vi "Get Segments.vi"(8 "error in (no error)":errorcluster, 9 "Pct-Encoded? (F)":bool, 11 "URI-Component.Path in":refnum<class "URI-Component.Path.lvclass">) -> (0 "error out":errorcluster, 2 "Segments":string[](array[string]), 3 "URI-Component.Path out":refnum<class "URI-Component.Path.lvclass">)   [LabVIEW 2013, in "openURI.lvlib" / "URI-Component.Path.lvclass"]
uses:
  URI-Component.Path.lvclass
  URI-Component.Path.lvclass/URI-Component.Path.ctl
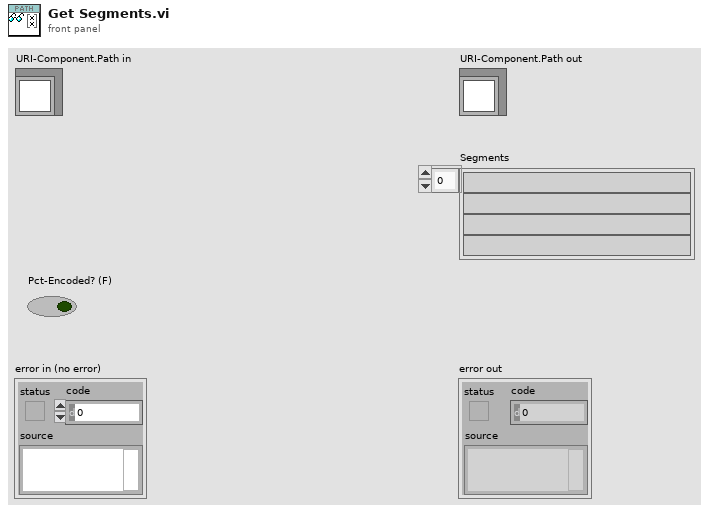
[diagram p1: front panel]
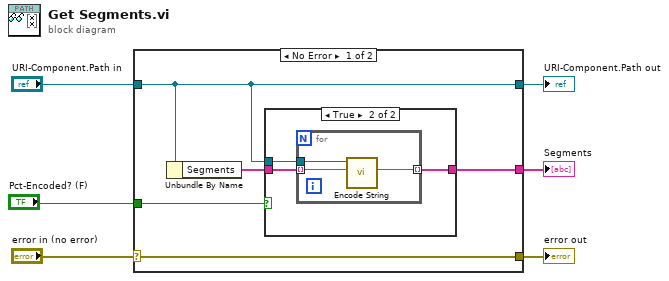
[diagram p0: block diagram]
diagram:
  n1 = case shown="No Error" "error in (no error)" {
    selector: "error in (no error)" -> [w11 w19]
    tunnel: [w11 w19] -> w5
    tunnel: [w7 w20] -> w3
    tunnel: "URI-Component.Path in" -> [w7 w20]
    tunnel: [w9 _] -> w2
    tunnel: "Pct-Encoded? (F)" -> [w8 _]
    frame No Error {
      n2 = Unbundle By Name(w7) -> ("Segments"=w10:string[])
      n3 = case shown="True" w8 {
        tunnel: w10 -> [w12 w15]
        tunnel: [w12 w14] -> w9
        tunnel: w7 -> [_ w13]
        frame False {
        }
        frame True {
          n4 = for {
            tunnel: w15 -> [w18] mode=indexing
            tunnel: [w17] -> w14 mode=indexing
            tunnel: w13 -> [w16]
            n5 = call-dynamic "Encode String.vi"("String"=w18, "URI-Component.Path"=w16) -> ("Encoded String"=w17:string)  [unwired: 9 in]
          }
        }
      }
    }
    frame Error {
    }
  }
  "error out" <- w5
  "URI-Component.Path out" <- w3
  "Segments" <- w2
